vi "Create linear LUT.vi"(7 "Input Image Type":T1 items=["Grayscale (U8)", "Grayscale (I16)", "Grayscale (SGL)", "Complex (CSG)", "RGB (U32)", "HSL (U32)", "RGB (U64)", "Grayscale (U16)"], 8 "White Value":dbl, 9 "Black Value":dbl) -> (0 "LUT (U8) Out":u8[](array[numeric]), 3 "Palette Out":cluster{"Red":u8, "Green":u8, "Blue":u8}[](array[cluster]))   [LabVIEW 2011]
doc: "Makes a linear LUT. Only valid modes of operation are 16 -> 8 and 8 -> 8 bits. The LUT is intended for use by IMAQ Vision routines and uses the indexing convention of that program, which is twos-complement signed for 16 bit images. This means that element 0 gives the value imput intensity 0, element 32,767 for int. 32,767, and el. 65536 for int. -1."
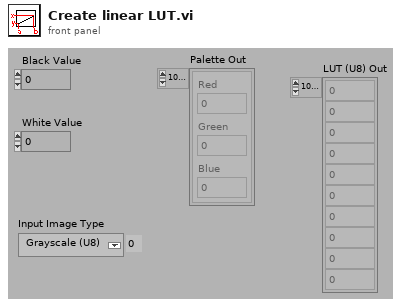
[diagram p1: front panel]
types:
  T1 = typedef "Image Type" = u32
  T2 = cluster{"upper limit":dbl, "upper limit":dbl, "upper limit":dbl}
  T3 = cluster{"upper limit":dbl, "upper limit":dbl, "upper limit":dbl}[]
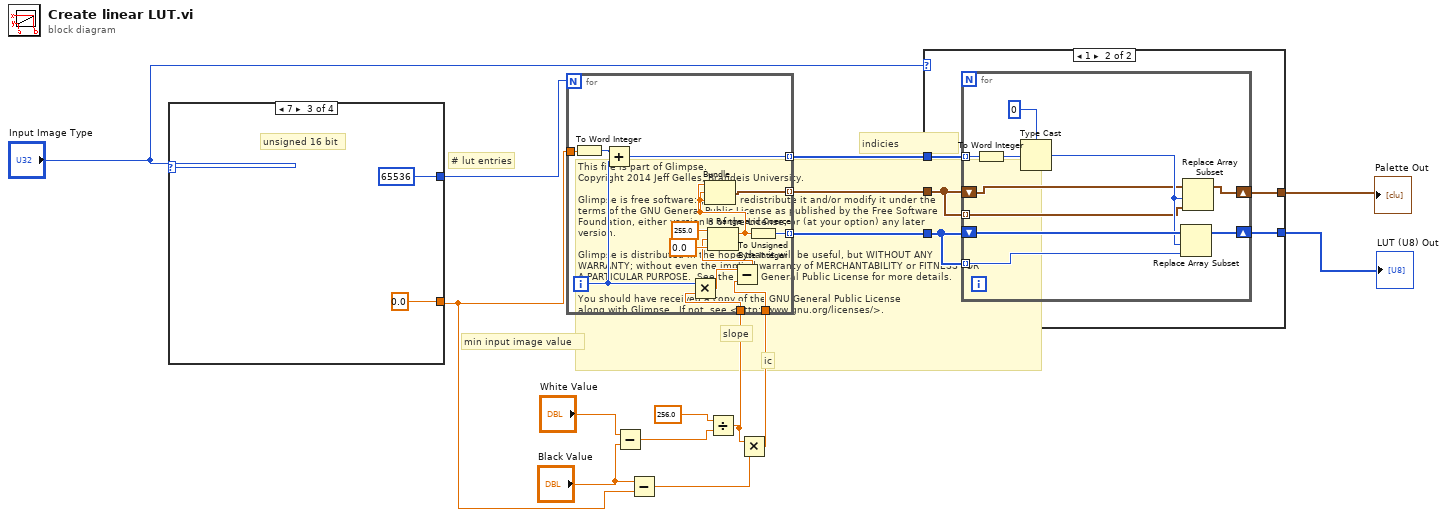
[diagram p0: block diagram]
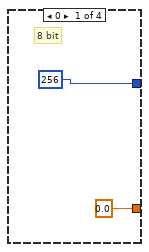
[diagram p3: hidden frame]
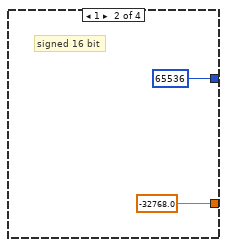
[diagram p4: hidden frame]
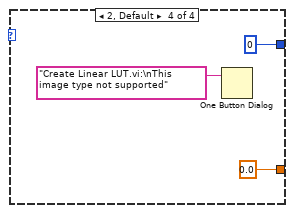
[diagram p5: hidden frame]
diagram:
  # "This file is part of Glimpse. \nCopyright 2014 Jeff Gelles, Brandeis University.    \n\nGlimpse is free software: you can redistribute it and/or modify it under the \nterms of the GNU General Public License as published by the Free Software \nFoundation, either version 3 of the License, or (at your option) any later \nversion.\n\nGlimpse is distributed in the hope that it will be useful, but WITHOUT ANY \nWARRANTY; without even the implied warranty of MERCHANTABILITY or FITNESS FOR \nA PARTICULAR PURPOSE.  See the GNU General Public License for more details.\n\nYou should have received a copy of the GNU General Public License\nalong with Glimpse.  If not, see <http://www.gnu.org/licenses/>."
  # "indicies"
  # "min input image value"
  # "ic"
  # "slope"
  # "# lut entries"
  n1 = case shown="7" "Input Image Type" {
    tunnel: [256 65536 65536 0] -> w10
    tunnel: [0.0 -32768.0 0.0 0.0] -> w7
    frame 0 {
      # "8 bit"
    }
    frame 1 {
      # "signed 16 bit"
    }
    frame 7 {
      # "unsigned 16 bit"
    }
    frame 2, Default {
      n2 = One Button Dialog(message="Create Linear LUT.vi:\nThis image type not supported") -> ()  [unwired: 2 out]
    }
  }
  n3 = Subtract(x="White Value", y="Black Value") -> (x-y=w11:dbl)
  n4 = Subtract(x="Black Value", y=w7) -> (x-y=w8:dbl)
  n5 = Divide(x=256.0 ("t"), y=w11) -> (x/y=w12:dbl)
  n6 = Multiply(x=w12, y=w8) -> (x*y=w13:dbl)
  n7 = for {
    N: w10 -> [_]
    tunnel: w12 -> [w37]
    tunnel: w13 -> [w36]
    tunnel: [w32] -> w2 mode=indexing
    tunnel: [w30] -> w4 mode=indexing
    tunnel: w7 -> [w27]
    tunnel: [w26] -> w6 mode=indexing
    i -> [w28]
    n8 = To Word Integer(number=w27) -> (16bit integer=w25:i16)
    n9 = Add(x=w25, y=w28) -> (x+y=w26:i32)
    n10 = Multiply(x=w28, y=w37) -> (x*y=w35:dbl)
    n11 = Subtract(x=w35, y=w36) -> (x-y=w33:dbl)
    n12 = In Range and Coerce(upper limit=255.0, x=w33, lower limit=0.0) -> (coerced(x)=w31:dbl)  [unwired: 1 out]
    n13 = Bundle("upper limit"=w31, "upper limit"=w31, "upper limit"=w31) -> (w32:T2)  [unwired: 1 out]
    n14 = To Unsigned Byte Integer(number=w31) -> (unsigned 8bit integer=w30:u8)
  }
  n15 = case shown="1" "Input Image Type" {
    tunnel: w6 -> [_ w44]
    tunnel: w4 -> [w39 w43]
    tunnel: [w39 w42] -> w3
    tunnel: w2 -> [w38 w41]
    tunnel: [w38 w40] -> w1
    frame 0, Default {
    }
    frame 1 {
      n16 = for {
        tunnel: w44 -> [w52] mode=indexing
        shift-right: [w54] -> w42
        shift-left: w43 -> [w50]
        tunnel: w43 -> [w49] mode=indexing
        shift-right: [w45] -> w40
        shift-left: w41 -> [w46]
        tunnel: w41 -> [w47] mode=indexing
        n17 = To Word Integer(number=w52) -> (16bit integer=w51:i16)
        n18 = Type Cast(type=u16 0, x=w51) -> (*(type *) &x=w48:u16)
        n19 = Replace Array Subset(array=w50, new element=w49, index=w48) -> (w54:u8[])
        n20 = Replace Array Subset(array=w46, new element=w47, index=w48) -> (w45:T3)
      }
    }
  }
  "Palette Out" <- w1
  "LUT (U8) Out" <- w3
